vi "noteOutputDeal.vi"(11 "note in editor":string) -> (3 "note output":string)   [LabVIEW 2010]
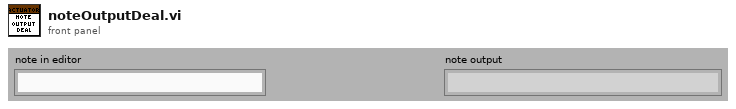
[diagram p1: front panel]
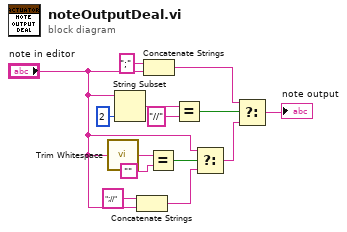
[diagram p0: block diagram]
diagram:
  n1 = call <vilib>:"Trim Whitespace.vi"("string"="note in editor") -> ("trimmed string"=w6:string)  [unwired: 1 in]
  n2 = String Subset(string="note in editor", length (rest)=2 ("length (rest)")) -> (substring=w13:string)  [unwired: 1 in]
  n3 = Concatenate Strings(";//" ("format string"), "note in editor") -> (w2:string)
  n4 = Concatenate Strings(";" ("string"), "note in editor") -> (w9:string)
  n5 = Equal?(x=w6, y="") -> (x = y?=w4:bool)
  n6 = Equal?(x=w13, y="//") -> (x = y?=w11:bool)
  n7 = Select(t="note in editor", s=w4, f=w2) -> (s? t:f=w1:string)
  n8 = Select(t=w9, s=w11, f=w1) -> (s? t:f=→"note output":string)
